vi "Checksum.vi"(11 "Data In":u8[](array[numeric]) format="%.0x") -> (2 "CkSum":u16 format="%.0x", 3 "Data with Cksum":u8[](array[numeric]) format="%.0x")   [LabVIEW 2018, in "EF20.lvlib" / "EF20.lvclass"]
uses:
  EF20.lvclass
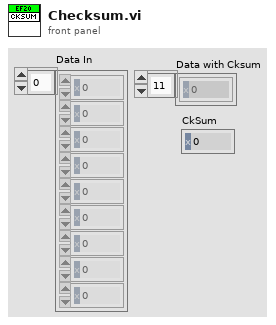
[diagram p1: front panel]
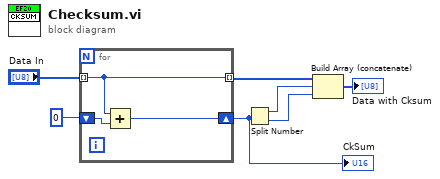
[diagram p0: block diagram]
diagram:
  n1 = for {
    tunnel: "Data In" -> [w8] mode=indexing
    shift-right: [w10] -> w5
    shift-left: u16 0 -> [w9]
    tunnel: [w8] -> w4 mode=indexing
    n2 = Add(x=w8, y=w9) -> (x+y=w10:u16)
  }
  "CkSum" <- w5
  n3 = Split Number(x=w5) -> (hi(x)=w3:u8, lo(x)=w2:u8)
  n4 = Build Array (concatenate)(w4, w3, w2) -> (→"Data with Cksum":u8[])
